vi "Get Windows Debug Options.vi"(8 "error in":errorcluster, 11 "data sharing framework custom device in":T1 format="%.0x") -> (0 "error out":errorcluster, 1 "show threads?":bool, 2 "show error dialog?":bool, 3 "data sharing framework custom device out":T1 format="%.0x")   [LabVIEW 2021, in "Data Sharing Framework Custom Device Scripting.lvlib"]
doc: "Reads the <b>show error dialog?</b> and <b>show threads?</b> options. These options are available for Windows targets."
uses:
  Data Sharing Framework Custom Device Scripting.lvlib
  Shared/DSF Shared.lvlib
  <vilib>/NI VeriStand/Custom Device API/Custom Device Item Ref.ctl
  <vilib>/NI VeriStand/Custom Device API/Custom Device API.lvlib
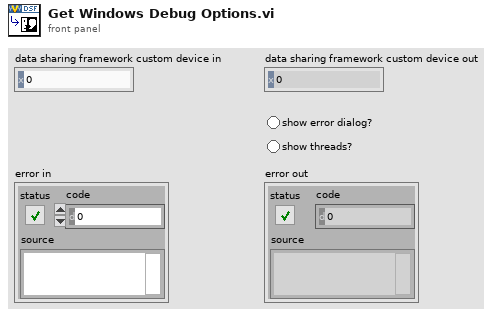
[diagram p1: front panel]
types:
  T1 = typedef "Custom Device API.lvlib/Custom Device Item Ref.ctl" = u64
  T2 = typedef "DSF Core.lvlibp/Framework.lvclass/Framework Options.ctl" = cluster{"FIFO Options":T3, "Thread Options":T4, "Plugin Options":T5, "Performance Options":T6, "Data Server Options":T7}
  T3 = typedef "DSF Core.lvlibp/Framework.lvclass/DSF FIFO Options.ctl" = cluster{"Infinite Timeouts":bool}
  T4 = typedef "DSF Core.lvlibp/Thread.lvclass/Thread Options.ctl" = cluster{"Show FP On Call":bool, "Close FP After Call":bool, "Allow Debugging":bool}
  T5 = typedef "DSF Core.lvlibp/Framework.lvclass/DSF Plugin Options.ctl" = cluster{"Default Components":bool}
  T6 = typedef "DSF Core.lvlibp/DSF Performance Options.ctl" = cluster{"Measure Period":bool, "Measure Rx/Tx Duration":bool}
  T7 = typedef "DSF Core.lvlibp/Framework.lvclass/Data Server Options.ctl" = cluster{"Enable Data Server":bool, "Period":u32}
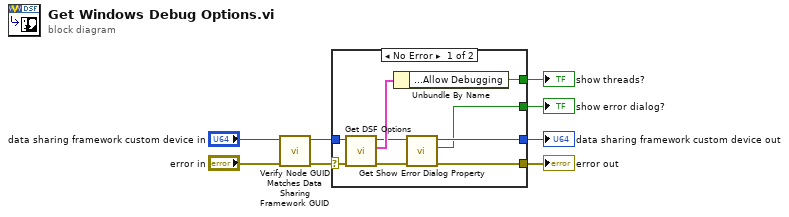
[diagram p0: block diagram]
diagram:
  n1 = call "Verify Node GUID Matches Data Sharing Framework GUID.vi"("error in"="error in", "data sharing framework custom device in"="data sharing framework custom device in") -> ("error out"=w1:errorcluster, "data sharing framework custom device out"=w2:T1)  [unwired: 8 in]
  n2 = case shown="No Error" w1 {
    selector: w1 -> [w9 w18]
    tunnel: [w16 _] -> w8
    tunnel: [w13 w18] -> w7
    tunnel: [w12 w19] -> w6
    tunnel: [w11 _] -> w5
    tunnel: w2 -> [w10 w19]
    frame No Error {
      n3 = call "Get DSF Options.vi"("error in (no error)"=w9, "Item Ref in"=w10) -> ("error out"=w14:errorcluster, "options"=w17:T2, "Item Ref out"=w15:T1)  [unwired: 7 in]
      n4 = Unbundle By Name(w17) -> ("Thread Options.Allow Debugging"=w16:bool)
      n5 = call "Get Show Error Dialog Property.vi"("error in (no error)"=w14, "Item Ref in"=w15) -> ("error out"=w13:errorcluster, "show error dialog"=w11:bool, "Item Ref out"=w12:T1)  [unwired: 7 in]
    }
    frame Error {
    }
  }
  "data sharing framework custom device out" <- w6
  "error out" <- w7
  "show threads?" <- w8
  "show error dialog?" <- w5
